vi "ProjectTest5.vi"() -> ()   [LabVIEW 2022 SP3]
uses:
  <vilib>/DAQmx/write.llb/DAQmx Write (Analog DBL 1Chan 1Samp).vi
  <vilib>/DAQmx/read.llb/DAQmx Read (Analog 1D DBL NChan 1Samp).vi
  <vilib>/DAQmx/write.llb/DAQmx Write (Digital 1D Bool 1Chan 1Samp).vi
  <vilib>/DAQmx/write.llb/DAQmx Write (Digital Bool 1Line 1Point).vi
  <vilib>/DAQmx/create/channels.llb/DAQmx Create Channel (AI-Voltage-Basic).vi
  <vilib>/DAQmx/create/channels.llb/DAQmx Create Channel (DO-Digital Output).vi
  <vilib>/DAQmx/create/channels.llb/DAQmx Create Channel (AO-Voltage-Basic).vi
  <vilib>/DAQmx/miscellaneous.llb/DAQmx Fill In Error Info.vi
  <vilib>/httpClient/PUTBuffer.vi
  <vilib>/httpClient/LabVIEWHTTPClient.lvlib
  <vilib>/ptbypt/NI_PtbyPt.lvlib
panel:
  out "Waveform Chart":dbl(graph)
  out "Light":bool
  out "MainFoodStorageLevel":dbl
  out "Main Food Container Level":string
  in  "MainFoodStorage":cluster{"MainFoodLevel":dbl}
  out "MainFoodLevel":sgl(slide) scale=10000.0..12000.0
  out "Buzzer Signal":string
  out "Buzzer":cluster{"Enable":bool}
  in  "DC Motor Speed":dbl(knob) scale=0.0..10.0
  in  "Buzzer Control":tag
  in  "Turn On the Light":tag
  out "Portion Size":string
  out "FoodPortion":cluster{"PortionSize":dbl}
  in  "DC Motor Control":tag
  out "Bowl Weight":dbl
  in  "stop 2":bool
  in  "Load Cell for Bowl Weight \nLDR for Night Detection (To Turn On Light)\nCustom Sensor for Main Food Storage Level":tag
  out "FeedNow Command":string
  out "Feed":cluster{"FeedNow":bool}
  # "SMART PET FEEDER"
  # "Feed Command, Food Portion and DC Motor Control"
  # "Main Food Storage Level"
  # "Night Light"
  # "Buzzer Control"
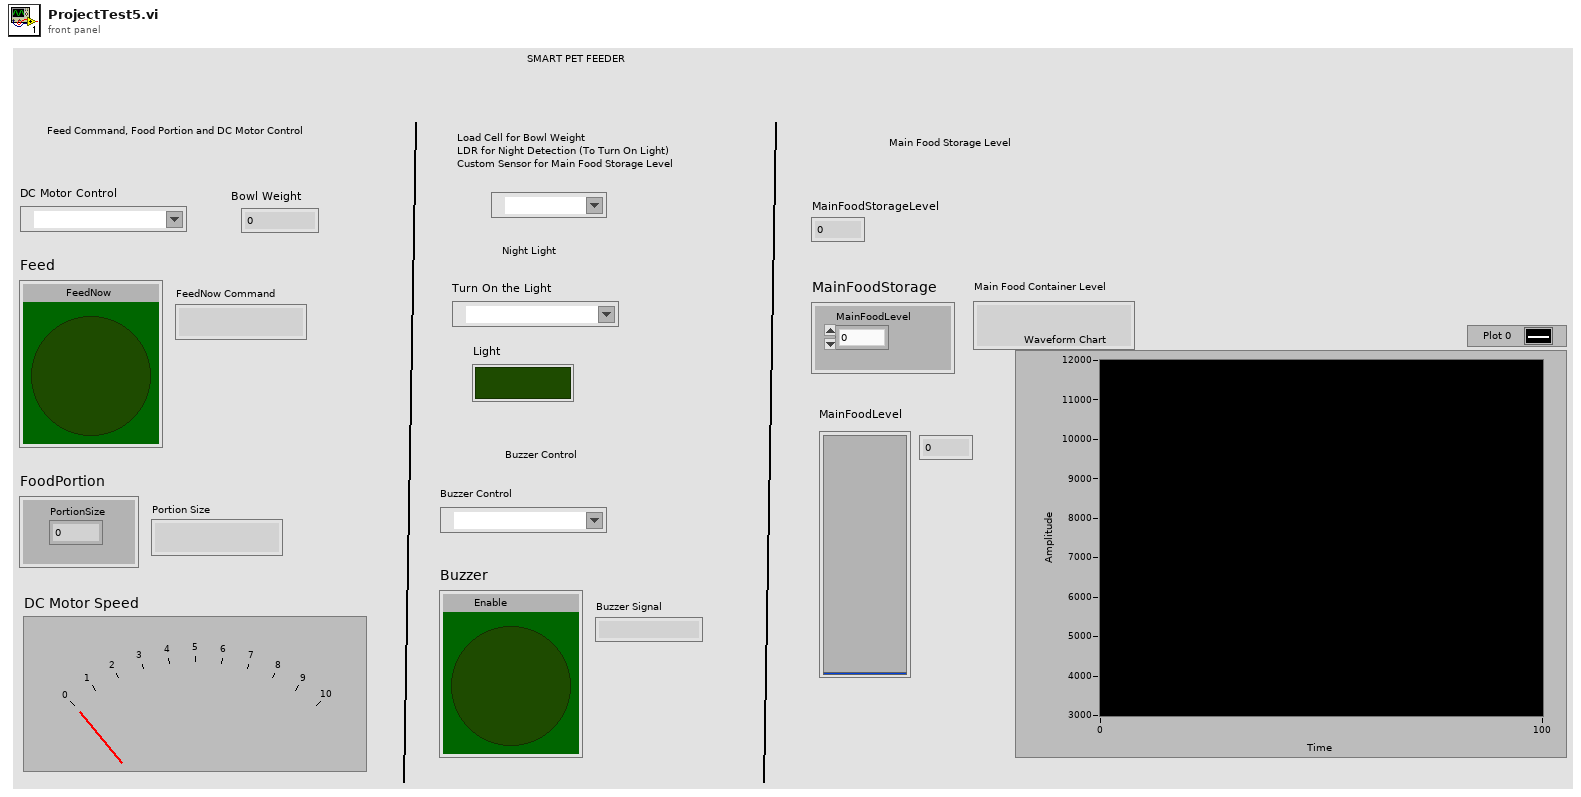
[diagram p1: front panel]
types:
  T1 = typedef "LabVIEWHTTPClient.lvlib/ClientHandle.ctl" = refnum<k1>
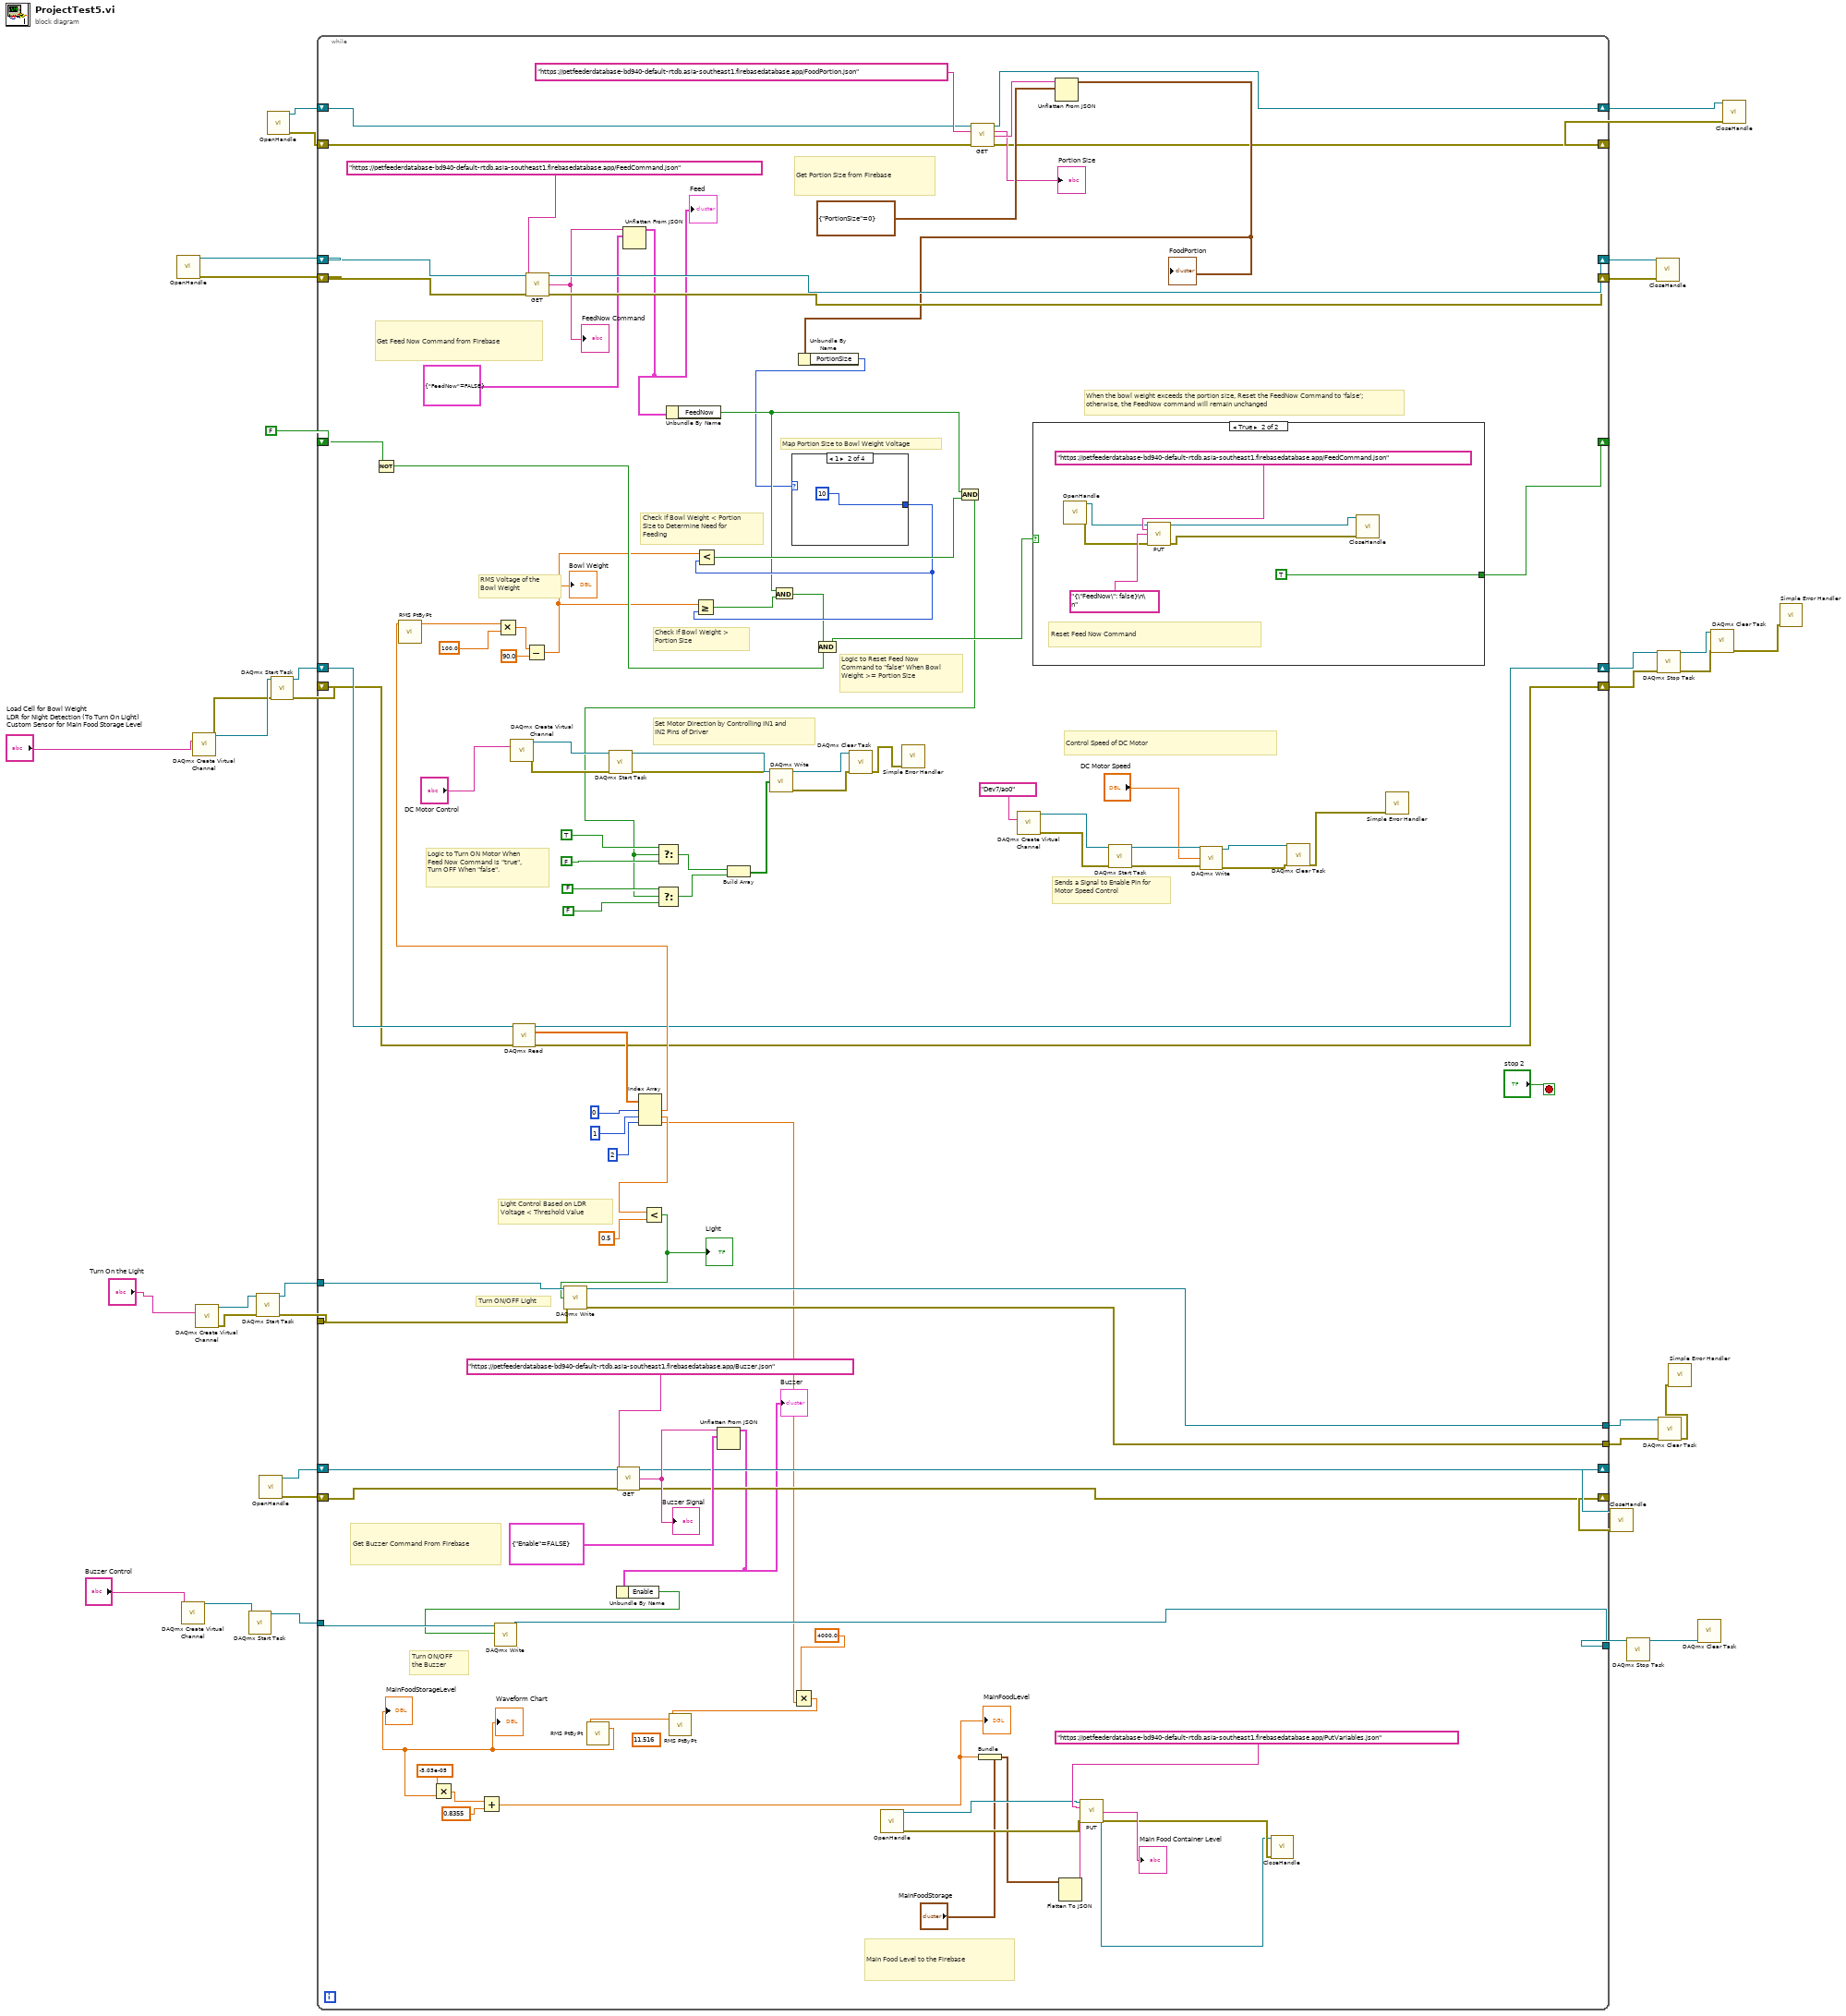
[diagram p0: block diagram]
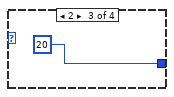
[diagram p4: hidden frame]
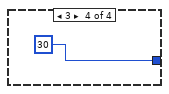
[diagram p5: hidden frame]
diagram:
  n1 = call <vilib>:"OpenHandle.vi"() -> ("client handle out"=w36:T1, "error out"=w34:errorcluster)  [unwired: 14 in]
  n2 = call-poly <vilib>:"DAQmx Create Virtual Channel.vi"("lines"="Buzzer Control") -> ("task out"=w8:refnum<k21>)  [unwired: 13 in, 1 out]
  n3 = call-poly <vilib>:"DAQmx Create Virtual Channel.vi"("physical channels"="Load Cell for Bowl Weight \nLDR for Night Detection (To Turn On Light)\nCustom Sensor for Main Food Storage Level") -> ("task out"=w30:refnum<k21>, "error out"=w29:errorcluster)  [unwired: 13 in]
  n4 = call-poly <vilib>:"DAQmx Create Virtual Channel.vi"("lines"="Turn On the Light") -> ("task out"=w18:refnum<k21>, "error out"=w17:errorcluster)  [unwired: 13 in]
  n5 = call <vilib>:"DAQmx Start Task.vi"("task/channels in"=w8) -> ("task out"=w6:refnum<k21>)  [unwired: 13 in, 1 out]
  n6 = call <vilib>:"DAQmx Start Task.vi"("task/channels in"=w18, "error in"=w17) -> ("task out"=w14:refnum<k21>, "error out"=w13:errorcluster)  [unwired: 12 in]
  n7 = call <vilib>:"OpenHandle.vi"() -> ("client handle out"=w1:T1, "error out"=w2:errorcluster)  [unwired: 14 in]
  n8 = call <vilib>:"OpenHandle.vi"() -> ("client handle out"=w21:T1, "error out"=w20:errorcluster)  [unwired: 14 in]
  n9 = call <vilib>:"DAQmx Start Task.vi"("task/channels in"=w30, "error in"=w29) -> ("task out"=w23:refnum<k21>, "error out"=w22:errorcluster)  [unwired: 12 in]
  n10 = while {
    shift-right: [w137] -> w35
    shift-left: w36 -> [w138]
    shift-right: [w135] -> w33
    shift-left: w34 -> [w136]
    shift-right: [w123] -> _
    shift-left: FALSE -> [w128]
    shift-right: [w82] -> w25
    shift-left: w23 -> [w92]
    shift-right: [w81] -> w24
    shift-left: w22 -> [w89]
    shift-right: [w99] -> w28
    shift-left: w21 -> [w97]
    shift-right: [w98] -> w27
    shift-left: w20 -> [w96]
    tunnel: w14 -> [w88]
    tunnel: w13 -> [w87]
    tunnel: [w84] -> w11
    tunnel: [w83] -> w10
    tunnel: w6 -> [w72]
    tunnel: [w71] -> w5
    shift-right: [w64] -> w3
    shift-left: w2 -> [w63]
    shift-right: [w65] -> w4
    shift-left: w1 -> [w62]
    stop <- "stop 2" stop-if-true
    (unwired) 11.516 ("x")
    # "Turn ON/OFF Light"
    # "When the bowl weight exceeds the portion size, Reset the FeedNow Command to ‘false’; otherwise, the FeedNow command will remain unchanged"
    # "Map Portion Size to Bowl Weight Voltage"
    # "Main Food Level to the Firebase"
    # "Turn ON/OFF the Buzzer"
    # "Get Buzzer Command From Firebase"
    # "Light Control Based on LDR Voltage < Threshold Value"
    # "Set Motor Direction by Controlling IN1 and IN2 Pins of Driver"
    # "Sends a Signal to Enable Pin for Motor Speed Control"
    # "Control Speed of DC Motor"
    # "Logic to Turn ON Motor When Feed Now Command is \"true\", Turn OFF When \"false\"."
    # "Logic to Reset Feed Now Command to \"false\" When Bowl Weight >= Portion Size"
    # "Check if Bowl Weight > Portion Size"
    # "Check if Bowl Weight < Portion Size to Determine Need for Feeding"
    # "RMS Voltage of the Bowl Weight"
    # "Get Feed Now Command from Firebase"
    # "Get Portion Size from Firebase"
    n11 = Not(x=w128) -> (.not. x?=w125:bool)
    n12 = call-poly <vilib>:"DAQmx Create Virtual Channel.vi"("lines"="DC Motor Control") -> ("task out"=w112:refnum<k21>, "error out"=w111:errorcluster)  [unwired: 13 in]
    n13 = call-poly <vilib>:"DAQmx Read.vi"("task/channels in"=w92, "error in"=w89) -> ("task out"=w82:refnum<k21>, "data"=w93:dbl[], "error out"=w81:errorcluster)  [unwired: 11 in]
    n14 = call <vilib>:"GET.vi"("client handle"=w138, "url"="https://petfeederdatabase-bd940-default-rtdb.asia-southeast1.firebasedatabase.app/FeedCommand.json", "error in (no error)"=w136) -> ("client handle out"=w137:T1, "body"=w134:string, "error out"=w135:errorcluster)  [unwired: 9 in, 1 out]
    "FeedNow Command" <- w134
    n15 = call <vilib>:"DAQmx Start Task.vi"("task/channels in"=w112, "error in"=w111) -> ("task out"=w114:refnum<k21>, "error out"=w113:errorcluster)  [unwired: 12 in]
    n16 = call <vilib>:"GET.vi"("client handle"=w62, "url"="https://petfeederdatabase-bd940-default-rtdb.asia-southeast1.firebasedatabase.app/Buzzer.json", "error in (no error)"=w63) -> ("client handle out"=w65:T1, "body"=w67:string, "error out"=w64:errorcluster)  [unwired: 9 in, 1 out]
    "Buzzer Signal" <- w67
    n17 = Unflatten From JSON(JSON string=w134, type and defaults=cluster{"FeedNow":bool} {"FeedNow"=FALSE}) -> (value=w132:cluster{"FeedNow":bool})  [unwired: 5 in, 1 out]
    "Feed" <- w132
    n18 = Index Array(array=w93, index #1=0 ("index"), index #2=1 ("index"), index #3=2 ("index")) -> (element #1=w85:dbl, element #2=w86:dbl, element #3=w48:dbl)
    n19 = call <vilib>:"RMS PtByPt.vi"("x"=w85) -> ("rms value"=w95:dbl)  [unwired: 3 in, 1 out]
    n20 = Multiply(x=w95, y=100.0) -> (x*y=w43:dbl)
    n21 = Subtract(x=w43, y=90.0) -> (x-y=w42:dbl)
    "Bowl Weight" <- w42
    n22 = Less?(x=w86, y=0.5) -> (x < y?=w49:bool)
    "Light" <- w49
    n23 = call-poly <vilib>:"DAQmx Write.vi"("task/channels in"=w88, "data"=w49, "error in"=w87) -> ("task out"=w84:refnum<k21>, "error out"=w83:errorcluster)  [unwired: 10 in, 1 out]
    n24 = Unbundle By Name(w132) -> ("FeedNow"=w127:bool)
    n25 = Unflatten From JSON(JSON string=w67, type and defaults=cluster{"Enable":bool} {"Enable"=FALSE}) -> (value=w61:cluster{"Enable":bool})  [unwired: 5 in, 1 out]
    "Buzzer" <- w61
    n26 = Unbundle By Name(w61) -> ("Enable"=w60:bool)
    n27 = call-poly <vilib>:"DAQmx Write.vi"("task/channels in"=w72, "data"=w60) -> ("task out"=w71:refnum<k21>)  [unwired: 11 in, 2 out]
    n28 = Multiply(x=4000.0, y=w48) -> (x*y=w46:dbl)
    n29 = call <vilib>:"RMS PtByPt.vi"("x"=w46) -> ("rms value"=w45:dbl)  [unwired: 3 in, 1 out]
    n30 = call <vilib>:"RMS PtByPt.vi"("x"=w45) -> ("rms value"=w41:dbl)  [unwired: 3 in, 1 out]
    "MainFoodStorageLevel" <- w41
    "Waveform Chart" <- w41
    n31 = Multiply(x=-5.03e-05, y=w41) -> (x*y=w39:dbl)
    n32 = Add(x=w39, y=0.8355) -> (x+y=w37:dbl)
    "MainFoodLevel" <- w37
    n33 = call <vilib>:"OpenHandle.vi"() -> ("client handle out"=w52:T1, "error out"=w55:errorcluster)  [unwired: 14 in]
    n34 = call <vilib>:"GET.vi"("client handle"=w97, "url"="https://petfeederdatabase-bd940-default-rtdb.asia-southeast1.firebasedatabase.app/FoodPortion.json", "error in (no error)"=w96) -> ("client handle out"=w99:T1, "headers"=→"Portion Size":string, "body"=w104:string, "error out"=w98:errorcluster)  [unwired: 9 in]
    n35 = Bundle(cluster="MainFoodStorage", "MainFoodLevel"=w37) -> (w50:cluster{"MainFoodLevel":dbl})
    n36 = call-poly <vilib>:"DAQmx Create Virtual Channel.vi"("physical channels"=tag "Dev7/ao0") -> ("task out"=w77:refnum<k21>, "error out"=w76:errorcluster)  [unwired: 13 in]
    n37 = Unflatten From JSON(JSON string=w104, type and defaults=cluster{"PortionSize":i32} {"PortionSize"=0}) -> (value=w101:cluster{"PortionSize":i32})  [unwired: 5 in, 1 out]
    "FoodPortion" <- w101
    n38 = Unbundle By Name(w101) -> ("PortionSize"=w100:i32)
    n39 = case shown="1" w100 {
      selector: w100 -> [w148 _ _ _]
      tunnel: [w148 10 20 30] -> w130
      frame 0, Default {
      }
      frame 1 {
      }
      frame 2 {
      }
      frame 3 {
      }
    }
    n40 = Greater Or Equal?(x=w42, y=w130) -> (x >= y?=w126:bool)
    n41 = Less?(x=w42, y=w130) -> (x < y?=w131:bool)
    n42 = And(x=w127, y=w126) -> (x .and. y?=w124:bool)
    n43 = And(x=w125, y=w124) -> (x .and. y?=w122:bool)
    n44 = And(x=w127, y=w131) -> (x .and. y?=w106:bool)
    n45 = Select(t=TRUE, s=w106, f=FALSE) -> (s? t:f=w117:bool)
    n46 = Select(t=FALSE, s=w106, f=FALSE) -> (s? t:f=w116:bool)
    n47 = Build Array(w117, w116) -> (w115:bool[])
    n48 = call-poly <vilib>:"DAQmx Write.vi"("task/channels in"=w114, "data"=w115, "error in"=w113) -> ("task out"=w109:refnum<k21>, "error out"=w108:errorcluster)  [unwired: 10 in, 1 out]
    n49 = call <vilib>:"DAQmx Clear Task.vi"("task in"=w109, "error in"=w108) -> ("error out"=w107:errorcluster)  [unwired: 13 in]
    n50 = call <vilib>:"Simple Error Handler.vi"("error in (no error)"=w107) -> ()  [unwired: 4 in, 5 out]
    n51 = case shown="True" w122 {
      selector: w122 -> [w140 _]
      tunnel: [w140 TRUE] -> w123
      frame False {
      }
      frame True {
        # "Reset Feed Now Command"
        n52 = call <vilib>:"OpenHandle.vi"() -> ("client handle out"=w144:T1, "error out"=w143:errorcluster)  [unwired: 14 in]
        n53 = call-poly <vilib>:"PUT.vi"("client handle"=w144, "url"="https://petfeederdatabase-bd940-default-rtdb.asia-southeast1.firebasedatabase.app/FeedCommand.json", "buffer"="{\"FeedNow\": false}\n\n", "error in (no error)"=w143) -> ("client handle out"=w142:T1, "error out"=w141:errorcluster)  [unwired: 8 in, 2 out]
        n54 = call <vilib>:"CloseHandle.vi"("client handle"=w142, "error in (no error)"=w141) -> ()  [unwired: 13 in, 1 out]
      }
    }
    n55 = Flatten To JSON(anything=w50) -> (JSON string=w56:string)  [unwired: 2 in, 1 out]
    n56 = call-poly <vilib>:"PUT.vi"("client handle"=w52, "url"="https://petfeederdatabase-bd940-default-rtdb.asia-southeast1.firebasedatabase.app/PutVariables.json", "buffer"=w56, "error in (no error)"=w55) -> ("client handle out"=w53:T1, "body"=→"Main Food Container Level":string, "error out"=w54:errorcluster)  [unwired: 8 in, 1 out]
    n57 = call <vilib>:"DAQmx Start Task.vi"("task/channels in"=w77, "error in"=w76) -> ("task out"=w80:refnum<k21>, "error out"=w79:errorcluster)  [unwired: 12 in]
    n58 = call-poly <vilib>:"DAQmx Write.vi"("task/channels in"=w80, "data"="DC Motor Speed", "error in"=w79) -> ("task out"=w74:refnum<k21>, "error out"=w73:errorcluster)  [unwired: 10 in, 1 out]
    n59 = call <vilib>:"CloseHandle.vi"("client handle"=w53, "error in (no error)"=w54) -> ()  [unwired: 13 in, 1 out]
    n60 = call <vilib>:"DAQmx Clear Task.vi"("task in"=w74, "error in"=w73) -> ("error out"=w75:errorcluster)  [unwired: 13 in]
    n61 = call <vilib>:"Simple Error Handler.vi"("error in (no error)"=w75) -> ()  [unwired: 4 in, 5 out]
  }
  n62 = call <vilib>:"CloseHandle.vi"("client handle"=w4, "error in (no error)"=w3) -> ()  [unwired: 13 in, 1 out]
  n63 = call <vilib>:"DAQmx Stop Task.vi"("task/channels in"=w5) -> ("task out"=w7:refnum<k21>)  [unwired: 13 in, 1 out]
  n64 = call <vilib>:"CloseHandle.vi"("client handle"=w35, "error in (no error)"=w33) -> ()  [unwired: 13 in, 1 out]
  n65 = call <vilib>:"DAQmx Stop Task.vi"("task/channels in"=w25, "error in"=w24) -> ("task out"=w19:refnum<k21>, "error out"=w26:errorcluster)  [unwired: 12 in]
  n66 = call <vilib>:"DAQmx Clear Task.vi"("task in"=w11, "error in"=w10) -> ("error out"=w12:errorcluster)  [unwired: 13 in]
  n67 = call <vilib>:"Simple Error Handler.vi"("error in (no error)"=w12) -> ()  [unwired: 4 in, 5 out]
  n68 = call <vilib>:"DAQmx Clear Task.vi"("task in"=w7) -> ()  [unwired: 14 in, 1 out]
  n69 = call <vilib>:"DAQmx Clear Task.vi"("task in"=w19, "error in"=w26) -> ("error out"=w31:errorcluster)  [unwired: 13 in]
  n70 = call <vilib>:"CloseHandle.vi"("client handle"=w28, "error in (no error)"=w27) -> ()  [unwired: 13 in, 1 out]
  n71 = call <vilib>:"Simple Error Handler.vi"("error in (no error)"=w31) -> ()  [unwired: 4 in, 5 out]
